vi "solar_cfg Variant to String.vi"(6 "ArrayDelimiters (1D,2D)":string[](array[string]), 8 "error in (no error)":errorcluster, 9 "Boolean as 0,1? (F)":bool, 10 "Use Enum Names? (F)":bool, 11 "Variant":variant) -> (0 "error out":errorcluster, 1 "Enum Names":string[](array[string]), 2 "Quotes Recommended?":bool, 3 "String":string)   [LabVIEW 2018]
doc: "This converts a <b>Variant</b> to ASCII <b>String</b>. To return enum names, set <b>User Enum Names?</b> to true. To return booleans as 0 or 1, set <b>Boolean as 0,1?</b> to true."
uses:
  <vilib>/Utility/Data Type/NI_Data Type.lvlib
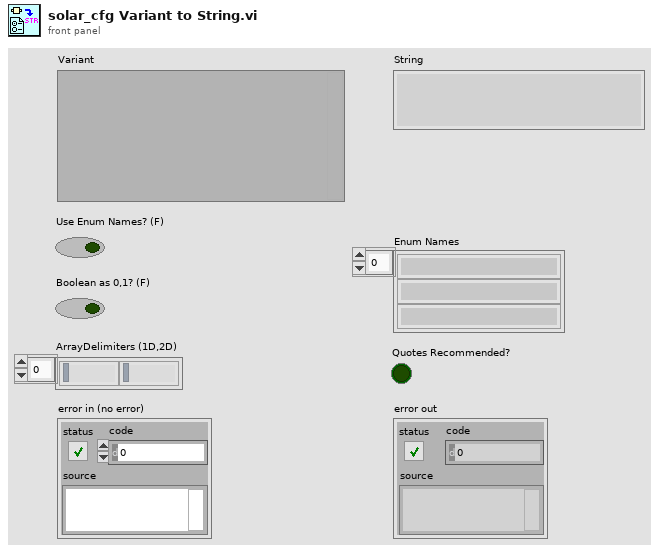
[diagram p1: front panel]
types:
  T1 = typedef "NI_Data Type.lvlib/Data Type.ctl" = enum8{"Invalid Type", "Void", "I8", "I16", "I32", "I64", "U8", "U16", "U32", "U64", "Single Float", "Double Float", "Extended Float", "Single Complex", "Double Complex", "Extended Complex", "Enum U8", "Enum U16", "Enum U32", "Enum U64", "Single Float With Unit", "Double Float With Unit", "Extended Float With Unit", "Single Complex with Unit", "Double Complex with Unit", "Extended Complex with Unit", "Boolean", "String", "Path", "Picture", "Tag", "Array", "Cluster", "Variant", "LV Variant", "Waveform", "Timestamp", "Digital Waveform", "Digital Data", "ExpressData", "Refnum", "External Data", "VI", "Poly VI", "LabVIEW Class Instance", "Fixed Point", "Set Collection", "Map Collection"}
  T2 = typedef "NI_Data Type.lvlib/Refnum Type.ctl" = enum16{"NotARefnum", "UnknownRefnum", "Generic", "Datalog", "ByteStream", "Device", "Occurence", "TCPNetConnection", "Auto", "Menu", "Imaq", "Hardware", "DataSocket", "Visa", "IVI", "UDPNetConnection", "Notifier", "Queue", "Irda", "EventReg", "DotNet", "UserEvent", "Callback", "UNUSED_EMPTY_POSITION", "BlueToothNetConnection", "LVObjApp", "LVObjVI", "LVObjUnknown", "GenericClass", "UserDefinedRefnumTag", "DataValue", "RT FIFO", "TDMS File", "PythonSessionRefnum"}
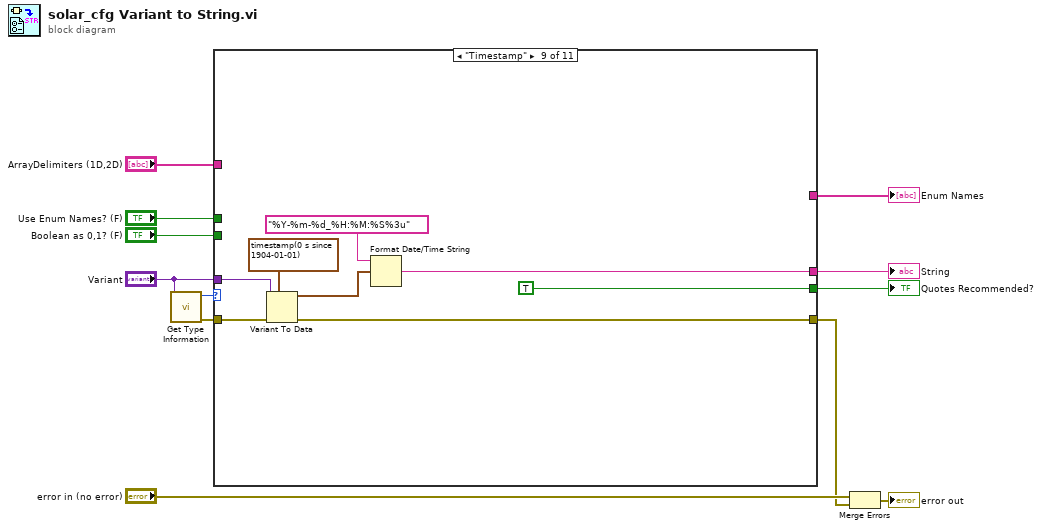
[diagram p0: block diagram]
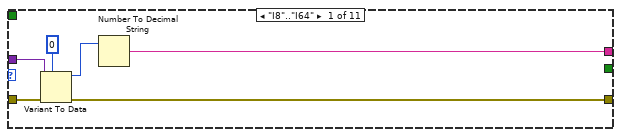
[diagram p2: hidden frame]
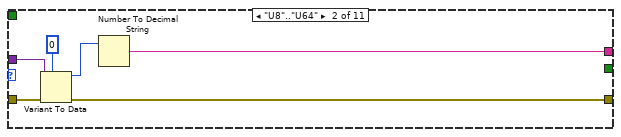
[diagram p3: hidden frame]
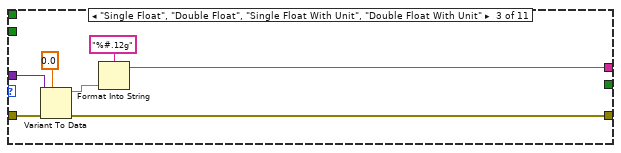
[diagram p4: hidden frame]
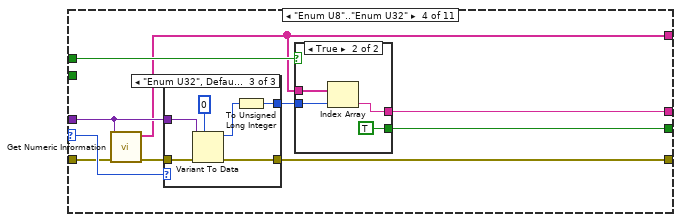
[diagram p5: hidden frame]
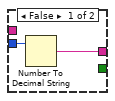
[diagram p6: hidden frame]
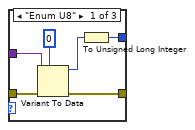
[diagram p7: hidden frame]
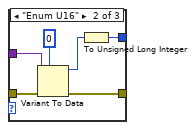
[diagram p8: hidden frame]
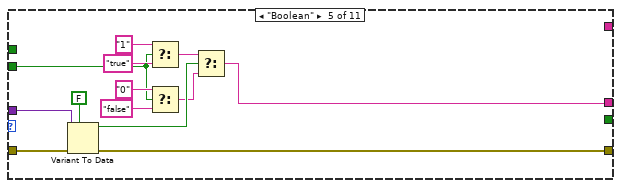
[diagram p9: hidden frame]
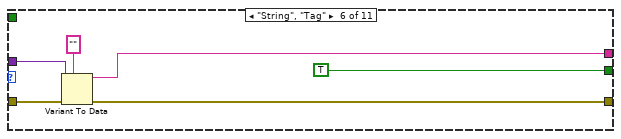
[diagram p10: hidden frame]
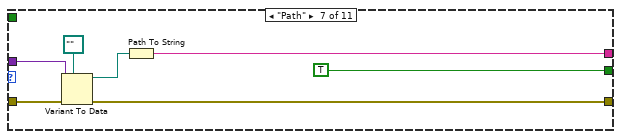
[diagram p11: hidden frame]
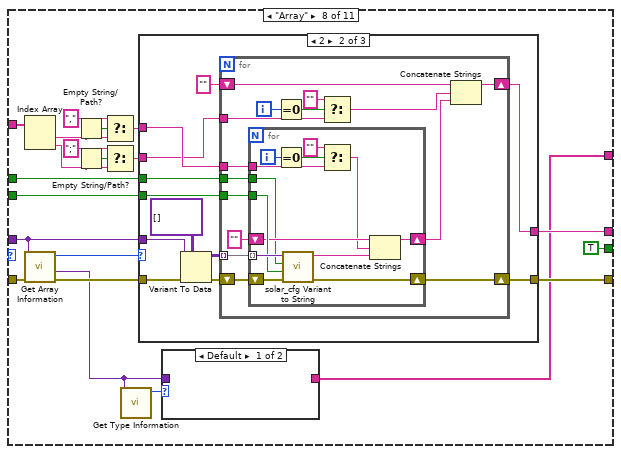
[diagram p12: hidden frame]
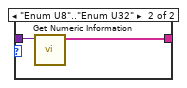
[diagram p13: hidden frame]
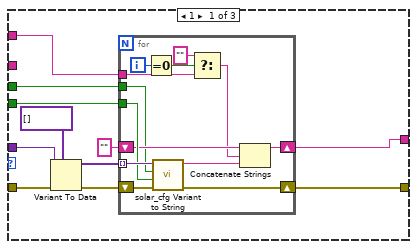
[diagram p14: hidden frame]
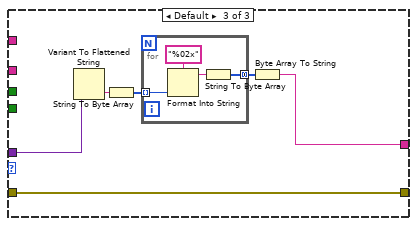
[diagram p15: hidden frame]
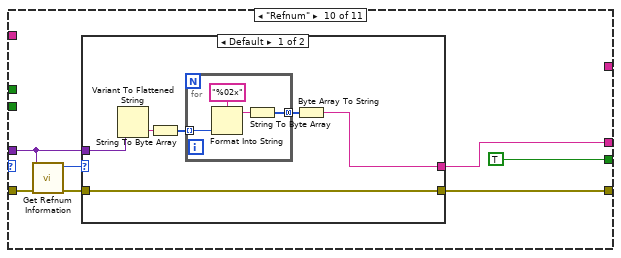
[diagram p16: hidden frame]
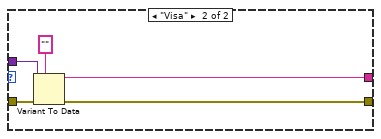
[diagram p17: hidden frame]
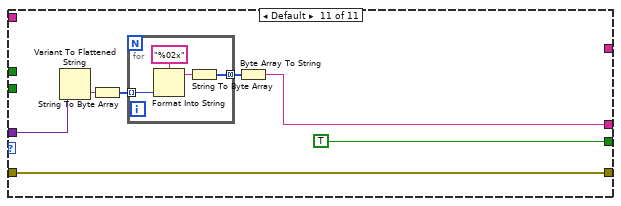
[diagram p18: hidden frame]
diagram:
  n1 = call <vilib>:"Get Type Information.vi"("variant"="Variant") -> ("error out"=w11:errorcluster, "type"=w12:T1)  [unwired: 6 in, 3 out]
  n2 = case shown="\"Timestamp\"" w12 {
    selector: w12 -> [_ _ _ w38 _ _ _ _ _ _ _]
    tunnel: "Variant" -> [w17 w23 w30 w36 w69 w83 w90 w109 w195 w200 w221]
    tunnel: w11 -> [w18 w24 w31 w37 w70 w84 w91 w112 w196 w201 w225]
    tunnel: [w15 w21 w28 w41 w66 w81 w88 w98 w194 w203 w225] -> w2
    tunnel: [w13 w19 w26 w39 w67 w80 w86 w97 w191 w202 w220] -> w9
    tunnel: "Boolean as 0,1? (F)" -> [_ _ _ _ w68 _ _ w101 _ _ _]
    tunnel: [_ _ _ w33 _ _ _ w92 _ _ _] -> w8
    tunnel: "Use Enum Names? (F)" -> [_ _ _ w34 _ _ _ w100 _ _ _]
    tunnel: [_ _ _ w32 _ TRUE TRUE TRUE TRUE TRUE TRUE] -> w5
    tunnel: "ArrayDelimiters (1D,2D)" -> [_ _ _ _ _ _ _ w106 _ _ _]
    frame "I8".."I64" {
      n3 = Variant To Data(error in=w18, type=i64 0, Variant=w17) -> (data=w14:i64, error out=w15:errorcluster)
      n4 = Number To Decimal String(number=w14) -> (decimal integer string=w13:string)  [unwired: 1 in]
    }
    frame "U8".."U64" {
      n5 = Variant To Data(error in=w24, type=u64 0, Variant=w23) -> (data=w20:u64, error out=w21:errorcluster)
      n6 = Number To Decimal String(number=w20) -> (decimal integer string=w19:string)  [unwired: 1 in]
    }
    frame "Single Float", "Double Float", "Single Float With Unit", "Double Float With Unit" {
      n7 = Variant To Data(error in=w31, type=0.0, Variant=w30) -> (data=w27:dbl, error out=w28:errorcluster)
      n8 = Format Into String(format string="%#.12g", w27) -> (resulting string=w26:string)  [unwired: 2 in, 1 out]
    }
    frame "Enum U8".."Enum U32" {
      n9 = call <vilib>:"Get Numeric Information.vi"("error in (no error)"=w37, "variant"=w36) -> ("error out"=w35:errorcluster, "enum names"=w33:string[])  [unwired: 6 in, 2 out]
      n10 = case shown="\"Enum U32\", Default" w38 {
        tunnel: w35 -> [w53 w59 w65]
        tunnel: w36 -> [w52 w58 w64]
        tunnel: [w50 w56 w62] -> w41
        tunnel: [w48 w54 w60] -> w40
        frame "Enum U8" {
          n11 = Variant To Data(error in=w53, type=u8 0, Variant=w52) -> (data=w49:u8, error out=w50:errorcluster)
          n12 = To Unsigned Long Integer(number=w49) -> (unsigned 32bit integer=w48:u32)
        }
        frame "Enum U16" {
          n13 = Variant To Data(error in=w59, type=u16 0, Variant=w58) -> (data=w55:u16, error out=w56:errorcluster)
          n14 = To Unsigned Long Integer(number=w55) -> (unsigned 32bit integer=w54:u32)
        }
        frame "Enum U32", Default {
          n15 = Variant To Data(error in=w65, type=u32 0, Variant=w64) -> (data=w61:u32, error out=w62:errorcluster)
          n16 = To Unsigned Long Integer(number=w61) -> (unsigned 32bit integer=w60:u32)
        }
      }
      n17 = case shown="True" w34 {
        tunnel: w40 -> [w43 w47]
        tunnel: [w42 w45] -> w39
        tunnel: w33 -> [_ w46]
        tunnel: [_ TRUE] -> w32
        frame False {
          n18 = Number To Decimal String(number=w43) -> (decimal integer string=w42:string)  [unwired: 1 in]
        }
        frame True {
          n19 = Index Array(array=w46, index=w47) -> (element=w45:string)
        }
      }
    }
    frame "Boolean" {
      n20 = Variant To Data(error in=w70, type=FALSE, Variant=w69) -> (data=w77:bool, error out=w66:errorcluster)
      n21 = Select(t="1", s=w68, f="true") -> (s? t:f=w72:string)
      n22 = Select(t="0", s=w68, f="false") -> (s? t:f=w71:string)
      n23 = Select(t=w72, s=w77, f=w71) -> (s? t:f=w67:string)
    }
    frame "String", "Tag" {
      n24 = Variant To Data(error in=w84, type="", Variant=w83) -> (data=w80:string, error out=w81:errorcluster)
    }
    frame "Path" {
      n25 = Variant To Data(error in=w91, type=path "", Variant=w90) -> (data=w87:path, error out=w88:errorcluster)
      n26 = Path To String(path=w87) -> (string=w86:string)
    }
    frame "Array" {
      n27 = Index Array(array=w106) -> (element #1=w107:string, element #2=w105:string)  [unwired: 2 in]
      n28 = call <vilib>:"Get Array Information.vi"("error in (no error)"=w112, "variant"=w109) -> ("error out"=w110:errorcluster, "array element data type"=w93:variant, "number of dimensions"=w111:i32)  [unwired: 6 in, 1 out]
      n29 = Empty String/Path?(string/path=w107) -> (empty?=w108:bool)
      n30 = Empty String/Path?(string/path=w105) -> (empty?=w103:bool)
      n31 = Select(t=",", s=w108, f=w107) -> (s? t:f=w99:string)
      n32 = Select(t=";", s=w103, f=w105) -> (s? t:f=w95:string)
      n33 = call <vilib>:"Get Type Information.vi"("variant"=w93) -> ("type"=w94:T1)  [unwired: 6 in, 4 out]
      n34 = case shown="2" w111 {
        tunnel: w110 -> [w125 w150 w179]
        tunnel: w109 -> [w124 w149 w181]
        tunnel: w101 -> [w120 w145 _]
        tunnel: w100 -> [w119 w144 _]
        tunnel: w99 -> [w118 w143 _]
        tunnel: [w117 w142 w179] -> w98
        tunnel: [w115 w139 w180] -> w97
        tunnel: w95 -> [_ w141 _]
        frame 1 {
          n35 = Variant To Data(error in=w125, type=variant[] [], Variant=w124) -> (data=w121:variant[], error out=w122:errorcluster)
          n36 = for {
            tunnel: w121 -> [w137] mode=indexing
            tunnel: w120 -> [w136]
            tunnel: w119 -> [w126]
            shift-right: [w134] -> w115
            shift-left: "" -> [w133]
            tunnel: w118 -> [w129]
            shift-right: [w132] -> w117
            shift-left: w122 -> [w138]
            i -> [w131]
            n37 = Equal To 0?(x=w131) -> (x = 0?=w130:bool)
            n38 = call "solar_cfg Variant to String.vi"("error in (no error)"=w138, "Boolean as 0,1? (F)"=w136, "Use Enum Names? (F)"=w126, "Variant"=w137) -> ("error out"=w132:errorcluster, "String"=w135:string)  [unwired: 4 in, 2 out]
            n39 = Select(t="", s=w130, f=w129) -> (s? t:f=w128:string)
            n40 = Concatenate Strings(w133, w128, w135) -> (w134:string)
          }
        }
        frame 2 {
          n41 = Variant To Data(error in=w150, type=variant[][] [], Variant=w149) -> (data=w146:variant[][], error out=w147:errorcluster)
          n42 = for {
            tunnel: w146 -> [w164] mode=indexing
            tunnel: w145 -> [w163]
            tunnel: w144 -> [w162]
            tunnel: w143 -> [w160]
            shift-right: [w159] -> w142
            shift-left: w147 -> [w165]
            tunnel: w141 -> [w155]
            shift-right: [w152] -> w139
            shift-left: "" -> [w151]
            i -> [w156]
            n43 = for {
              tunnel: w164 -> [w177] mode=indexing
              tunnel: w163 -> [w176]
              tunnel: w162 -> [w166]
              shift-right: [w174] -> w158
              shift-left: "" -> [w173]
              tunnel: w160 -> [w169]
              shift-right: [w172] -> w159
              shift-left: w165 -> [w178]
              i -> [w171]
              n44 = Equal To 0?(x=w171) -> (x = 0?=w170:bool)
              n45 = call "solar_cfg Variant to String.vi"("error in (no error)"=w178, "Boolean as 0,1? (F)"=w176, "Use Enum Names? (F)"=w166, "Variant"=w177) -> ("error out"=w172:errorcluster, "String"=w175:string)  [unwired: 4 in, 2 out]
              n46 = Select(t="", s=w170, f=w169) -> (s? t:f=w168:string)
              n47 = Concatenate Strings(w173, w168, w175) -> (w174:string)
            }
            n48 = Equal To 0?(x=w156) -> (x = 0?=w157:bool)
            n49 = Select(t="", s=w157, f=w155) -> (s? t:f=w153:string)
            n50 = Concatenate Strings(w151, w153, w158) -> (w152:string)
          }
        }
        frame Default {
          n51 = Variant To Flattened String(Variant=w181) -> (data string=w182:string)  [unwired: 1 out]
          n52 = String To Byte Array(string=w182) -> (unsigned byte array=w184:u8[])
          n53 = for {
            tunnel: w184 -> [w188] mode=indexing
            tunnel: [w185] -> w183 mode=concatenating
            n54 = Format Into String(format string="%02x" ("Format String"), w188) -> (resulting string=w186:string)  [unwired: 2 in, 1 out]
            n55 = String To Byte Array(string=w186) -> (unsigned byte array=w185:u8[])
          }
          n56 = Byte Array To String(unsigned byte array=w183) -> (string=w180:string)
        }
      }
      n57 = case shown="Default" w94 {
        tunnel: w93 -> [_ w114]
        tunnel: [_ w113] -> w92
        frame Default {
        }
        frame "Enum U8".."Enum U32" {
          n58 = call <vilib>:"Get Numeric Information.vi"("variant"=w114) -> ("enum names"=w113:string[])  [unwired: 7 in, 3 out]
        }
      }
    }
    frame "Timestamp" {
      n59 = Variant To Data(error in=w196, type=timestamp(0 s since 1904-01-01), Variant=w195) -> (data=w192:timestamp, error out=w194:errorcluster)
      n60 = Format Date/Time String(time format string (%c)="%Y-%m-%d_%H:%M:%S%3u", seconds (now)=w192) -> (date/time string=w191:string)  [unwired: 1 in]
    }
    frame "Refnum" {
      n61 = call <vilib>:"Get Refnum Information.vi"("error in (no error)"=w201, "variant"=w200) -> ("error out"=w199:errorcluster, "reference type"=w198:T2)  [unwired: 6 in, 2 out]
      n62 = case shown="Default" w198 {
        tunnel: [w209 w217] -> w203
        tunnel: [w204 w216] -> w202
        tunnel: w200 -> [w205 w215]
        tunnel: w199 -> [w209 w214]
        frame Default {
          n63 = Variant To Flattened String(Variant=w205) -> (data string=w206:string)  [unwired: 1 out]
          n64 = String To Byte Array(string=w206) -> (unsigned byte array=w208:u8[])
          n65 = for {
            tunnel: w208 -> [w213] mode=indexing
            tunnel: [w210] -> w207 mode=concatenating
            n66 = Format Into String(format string="%02x" ("Format String"), w213) -> (resulting string=w211:string)  [unwired: 2 in, 1 out]
            n67 = String To Byte Array(string=w211) -> (unsigned byte array=w210:u8[])
          }
          n68 = Byte Array To String(unsigned byte array=w207) -> (string=w204:string)
        }
        frame "Visa" {
          n69 = Variant To Data(error in=w214, type="", Variant=w215) -> (data=w216:string, error out=w217:errorcluster)
        }
      }
    }
    frame Default {
      n70 = Variant To Flattened String(Variant=w221) -> (data string=w222:string)  [unwired: 1 out]
      n71 = String To Byte Array(string=w222) -> (unsigned byte array=w224:u8[])
      n72 = for {
        tunnel: w224 -> [w229] mode=indexing
        tunnel: [w226] -> w223 mode=concatenating
        n73 = Format Into String(format string="%02x" ("Format String"), w229) -> (resulting string=w227:string)  [unwired: 2 in, 1 out]
        n74 = String To Byte Array(string=w227) -> (unsigned byte array=w226:u8[])
      }
      n75 = Byte Array To String(unsigned byte array=w223) -> (string=w220:string)
    }
  }
  "String" <- w9
  "Enum Names" <- w8
  "Quotes Recommended?" <- w5
  n76 = Merge Errors("error in (no error)", w2) -> (→"error out":errorcluster)
